vi "ALARM Check Errors.vi"(8 "error in (no error)":errorcluster, 9 "ALARM Q":refnum<queue>, 10 "Data REF":T1, 11 "Data Cluster":T2={"LOG REF"=refnum, "Writer Queue"=refnum, "Log Path"=path "", "UPS standby"=FALSE, "status code"=5001, "SP"=[], "Over Sens Status"=[]}) -> (0 "error out":errorcluster, 3 "Data Cluster out":T2={"LOG REF"=refnum, "Writer Queue"=refnum, "Log Path"=path "", "UPS standby"=FALSE, "status code"=5001, "SP"=[], "Over Sens Status"=[]})   [LabVIEW 2020, in "QCT ALARM.lvlib"]
uses:
  QCT ALARM.lvlib
  ALARM Configuration.ctl
  support/Message Queue/Message Cluster.ctl
  support/PCT Data REFs.ctl
  <instrlib>/PalmSens SDK for LabVIEW 5.10/PalmSens/MeasurementResults.ctl
  <instrlib>/PalmSens SDK for LabVIEW 5.10/PalmSens/LiveCurveResult.ctl
  support/PCT FGV CMD.ctl
  support/Message Queue/Message Queue.lvlib
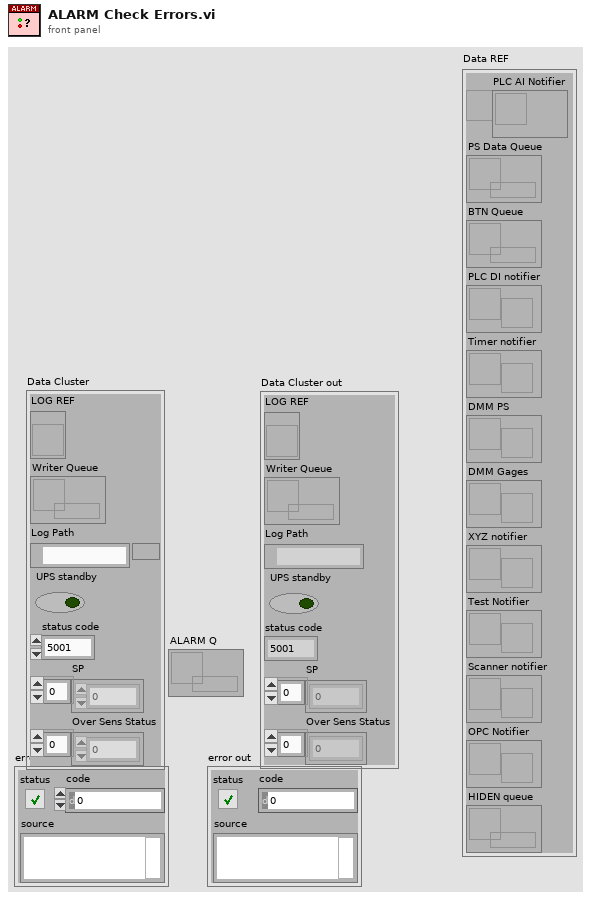
[diagram p1: front panel]
types:
  T1 = typedef "PCT Data REFs.ctl" = cluster{"PLC AI Notifier":refnum<notifier>, "PS Data Queue":refnum<queue>, "BTN Queue":refnum<queue>, "PLC DI notifier":refnum<notifier>, "Timer notifier":refnum<notifier>, "DMM PS":refnum<notifier>, "DMM Gages":refnum<notifier>, "XYZ notifier":refnum<notifier>, "Test Notifier":refnum<notifier>, "Scanner notifier":refnum<notifier>, "OPC Notifier":refnum<notifier>, "HIDEN queue":refnum<queue>}
  T2 = typedef "QCT ALARM.lvlib/ALARM Configuration.ctl" = cluster{"LOG REF":refnum<vi>, "Writer Queue":refnum<queue>, "Log Path":path, "UPS standby":bool, "status code":i32, "SP":dbl[], "Over Sens Status":dbl[]}
  T3 = typedef "PCT FGV CMD.ctl" = enum16{"INIT", "GET", "SET"}
  T4 = cluster{"Type CMD":string, "Mode CMD":string, "Main CMD":string}
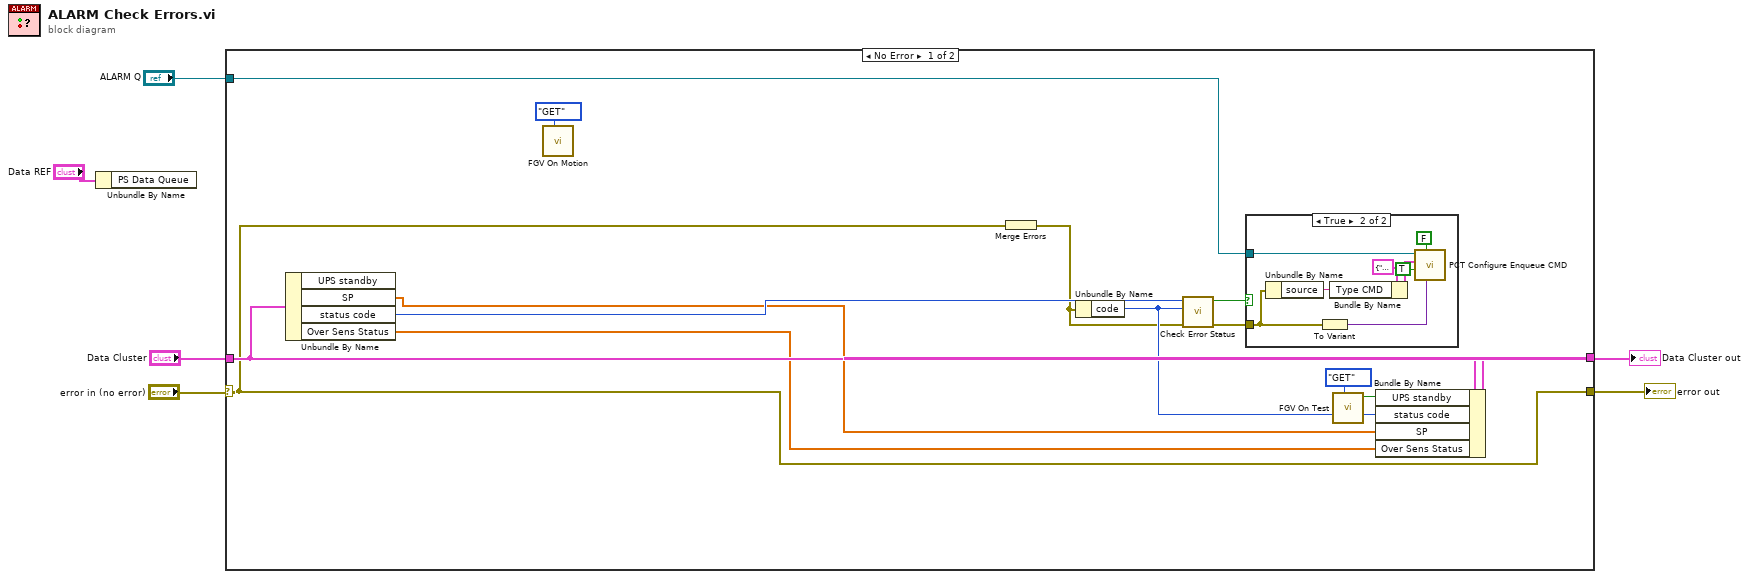
[diagram p0: block diagram]
diagram:
  n1 = Unbundle By Name("Data REF") -> ()  [unwired: 1 out]
  n2 = case shown="No Error" "error in (no error)" {
    selector: "error in (no error)" -> [w16 w29]
    tunnel: [w17 w30] -> w5
    tunnel: "Data Cluster" -> [w20 w30]
    tunnel: [w16 w29] -> w4
    tunnel: "ALARM Q" -> [w19 _]
    frame No Error {
      n3 = Unbundle By Name(w20) -> ("SP"=w12:dbl[], "status code"=w18:i32, "Over Sens Status"=w7:dbl[])  [unwired: 1 out]
      n4 = call "FGV On Motion.vi"("CMD"=PCT_FGV_CMD."GET") -> ()  [unwired: 9 in, 2 out]
      n5 = Merge Errors(w16) -> (w14:errorcluster)
      n6 = Unbundle By Name(w14) -> ("code"=w15:i32)
      n7 = call "Check Error Status.vi"("error in (no error)"=w14, "Current Code"=w15, "Previous Code"=w18) -> ("Error out"=w13:errorcluster, "Send Alarm"=w9:bool)  [unwired: 7 in]
      n8 = case shown="True" w9 {
        tunnel: w19 -> [_ w25]
        tunnel: w13 -> [_ w23]
        frame False {
        }
        frame True {
          n9 = Unbundle By Name(w23) -> ("source"=w22:string)
          n10 = To Variant(anything=w23) -> (Variant=w28:variant)
          n11 = Bundle By Name(cluster=T4 {"Type CMD"="", "Mode CMD"="", "Main CMD"="Error"} ("CMD"), "Type CMD"=w22) -> (w24:T4)
          n12 = call "PCT Configure Enqueue CMD.vi"("Parameter Data"=w28, "Read"=FALSE, "Priority Message? (F)"=TRUE, "CMD"=w24, "CMD Queue in"=w25) -> ()  [unwired: 4 in, 3 out]
        }
      }
      n13 = call "FGV On Test.vi"("CMD"=PCT_FGV_CMD."GET") -> ("output"=w11:bool)  [unwired: 9 in, 1 out]
      n14 = Bundle By Name(cluster=w20, "UPS standby"=w11, "status code"=w15, "SP"=w12, "Over Sens Status"=w7) -> (w17:T2)
    }
    frame Error {
    }
  }
  "error out" <- w4
  "Data Cluster out" <- w5
